vi "Refresh Channel Pairing.vi"(8 "error in (no error)":errorcluster, 10 "engine configuration in":refnum<class "engine configuration.lvclass">, 11 "E2E editor node in":refnum<class "E2E Tag Exchange editor node.lvclass">) -> (0 "error out":errorcluster, 2 "engine configuration out":refnum<class "engine configuration.lvclass">, 3 "E2E editor node out":refnum<class "E2E Tag Exchange editor node.lvclass">)   [LabVIEW 2015, in "E2E Tag Exchange editor node.lvclass"]
uses:
  E2E Tag Exchange editor node.lvclass
  <vilib>/NI/Module Execution Interface/Engine Configuration/engine configuration.lvclass
  E2E Tag Exchange editor node.lvclass/E2E Tag Exchange editor node.ctl
  module/configuration/E2E Tag Exchange configuration.lvclass/E2E Tag Exchange configuration.ctl
  <vilib>/NI/Configuration Framework/serializable configuration/NISE_CEF_serializable configuration.lvclass/NISE_CEF_serializable configuration.ctl
  module/configuration/Write Paired Module UID.vi
  module/configuration/Read Paired Module UID.vi
  <vilib>/Utility/LVClass/Get LV Class Name.vi
  <vilib>/NI/Configuration Framework/error generator/NISE_error generator.vi
  <vilib>/NI/DCAF/Tag Editor Core/Configuration Editor/Classes/Module editor node/module editor node.lvclass
  module/configuration/E2E Tag Exchange configuration.lvclass
  <vilib>/NI/Configuration Framework/serializable configuration/NISE_CEF_serializable configuration.lvclass
  <vilib>/NI/DCAF/Tag Editor Core/Configuration Editor/Classes/Engine Parent/Engine Parent Editor Node.lvclass
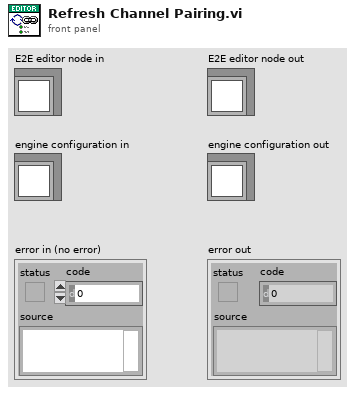
[diagram p1: front panel]
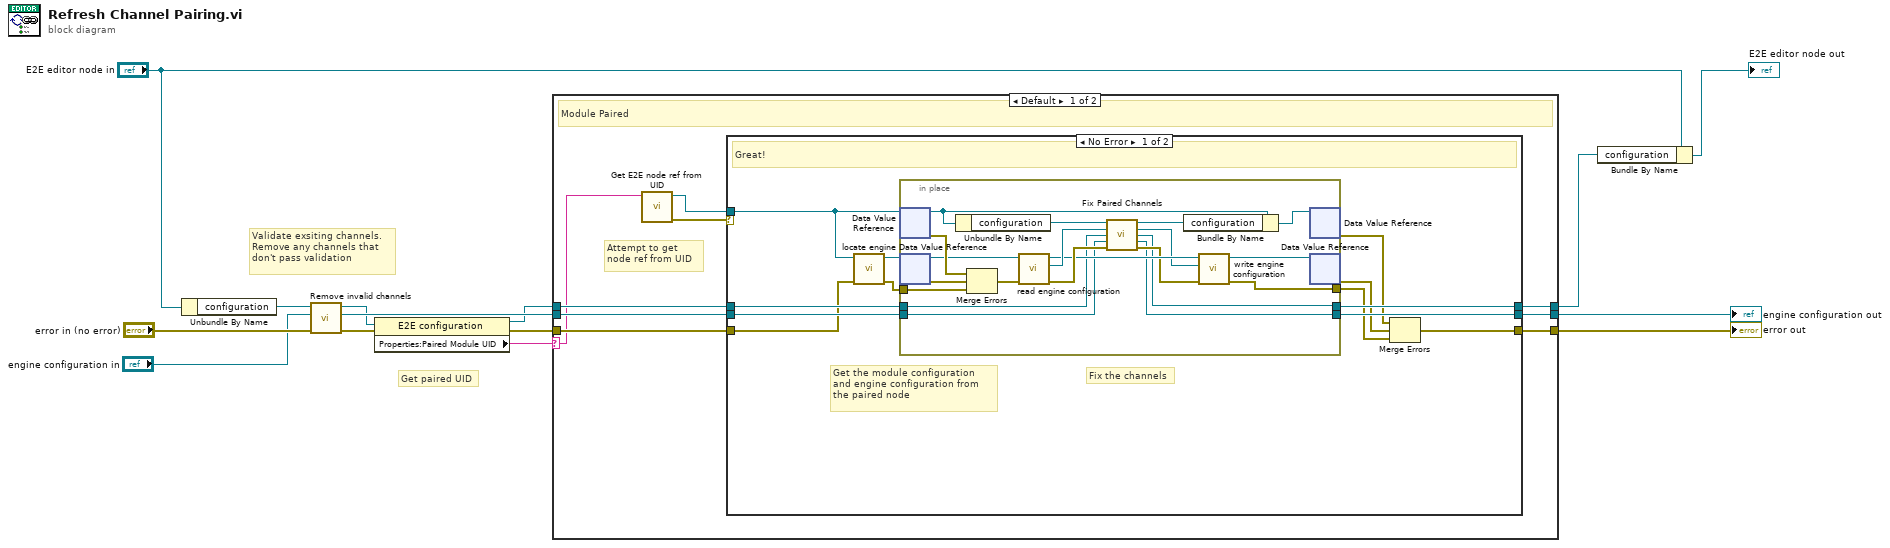
[diagram p0: block diagram]
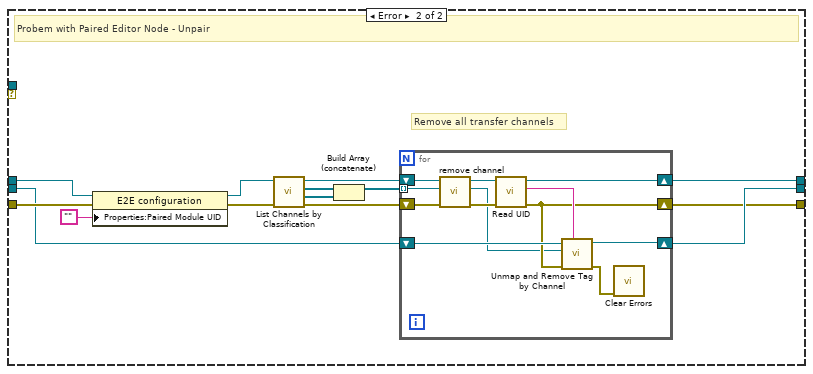
[diagram p2: hidden frame]
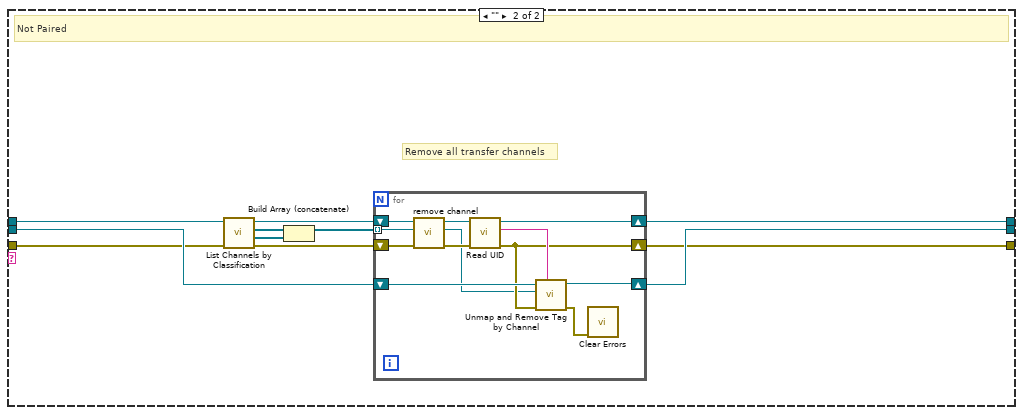
[diagram p3: hidden frame]
diagram:
  # "Get paired UID"
  # "Validate exsiting channels.\nRemove any channels that \ndon't pass validation"
  n1 = Unbundle By Name("E2E editor node in") -> ("configuration"=w14:refnum<class "E2E Tag Exchange configuration.lvclass">)
  n2 = call "Remove invalid channels.vi"("error in (no error)"="error in (no error)", "engine configuration in"="engine configuration in", "E2E configuration in"=w14) -> ("error out"=w11:errorcluster, "engine configuration out"=w8:refnum<class "engine configuration.lvclass">, "E2E configuration out"=w7:refnum<class "E2E Tag Exchange configuration.lvclass">)  [unwired: 6 in]
  n3 = property class="E2E configuration"(reference=w7, error in=w11) -> (reference out=w6:refnum<class "E2E Tag Exchange configuration.lvclass">, error out=w9:errorcluster, "Properties:Paired Module UID"=w10:string)
  n4 = case shown="Default" w10 {
    selector: w10 -> [w18 _]
    tunnel: w9 -> [w22 w81]
    tunnel: w8 -> [w20 w89]
    tunnel: w6 -> [w19 w85]
    tunnel: [w17 w87] -> w5
    tunnel: [w16 w88] -> w1
    tunnel: [w15 w86] -> w2
    frame Default {
      # "Attempt to get\nnode ref from UID"
      # "Module Paired"
      n5 = call "Get E2E node ref from UID.vi"("UID"=w18) -> ("error out"=w23:errorcluster, "E2E editor node ref"=w21:refnum<data-value>)  [unwired: 9 in]
      n6 = case shown="No Error" w23 {
        tunnel: w22 -> [w31 w68]
        tunnel: w21 -> [w33 _]
        tunnel: w20 -> [w35 w58]
        tunnel: w19 -> [w34 w67]
        tunnel: [w28 w56] -> w15
        tunnel: [w30 w60] -> w17
        tunnel: [w29 w57] -> w16
        frame No Error {
          # "Fix the channels"
          # "Get the module configuration\nand engine configuration from\nthe paired node"
          # "Great!"
          n7 = call <vilib>:"locate engine.vi"("error in"=w31, "component"=w33) -> ("error out"=w24:errorcluster, "engine"=w32:refnum<data-value>)  [unwired: 8 in]
          n8 = in-place {
            in-place-border: w35 -> [w41]
            in-place-border: w34 -> [w42]
            in-place-border: [w36] -> w27
            in-place-border: [w39] -> w30
            in-place-border: [w40] -> w29
            in-place-border: w24 -> [w55]
            n9 = in-place-dvr #1(w33) -> (w45:refnum<class "E2E Tag Exchange editor node.lvclass">, w53:errorcluster)
            n10 = in-place-dvr #2(w32) -> (w52:refnum<class "Engine Parent Editor Node.lvclass">, w54:errorcluster)
            n11 = Unbundle By Name(w45) -> ("configuration"=w49:refnum<class "E2E Tag Exchange configuration.lvclass">)
            n12 = Merge Errors(w53, w54, w55) -> (w51:errorcluster)
            n13 = call <vilib>:"read engine configuration.vi"("error in"=w51, "Engine Parent Editor Node in"=w52) -> ("error out"=w50:errorcluster, "engine configuration"=w48:refnum<class "engine configuration.lvclass">, "Engine Parent Editor Node out"=w47:refnum<class "Engine Parent Editor Node.lvclass">)  [unwired: 7 in]
            n14 = call "Fix Paired Channels.vi"("Paired E2E configuration in"=w49, "Paired engine configuration in"=w48, "E2E configuration in"=w42, "engine configuration in"=w41, "error in (no error)"=w50) -> ("Paired E2E configuration out"=w44:refnum<class "E2E Tag Exchange configuration.lvclass">, "Paired engine configuration out"=w46:refnum<class "engine configuration.lvclass">, "E2E configuration out"=w39:refnum<class "E2E Tag Exchange configuration.lvclass">, "engine configuration out"=w40:refnum<class "engine configuration.lvclass">, "error out"=w43:errorcluster)  [unwired: 6 in]
            n15 = Bundle By Name(cluster=w45, "configuration"=w44) -> (w38:refnum<class "E2E Tag Exchange editor node.lvclass">)
            n16 = call <vilib>:"write engine configuration.vi"("error in"=w43, "engine configuration"=w46, "Engine Parent Editor Node in"=w47) -> ("error out"=w36:errorcluster, "Engine Parent Editor Node out"=w37:refnum<class "Engine Parent Editor Node.lvclass">)  [unwired: 7 in]
            n17 = in-place-dvr #1(w38) -> (w25:errorcluster)  [unwired: 1 out]
            n18 = in-place-dvr #2(w37) -> (w26:errorcluster)  [unwired: 1 out]
          }
          n19 = Merge Errors(w25, w26, w27) -> (w28:errorcluster)
        }
        frame Error {
          # "Remove all transfer channels"
          # "Probem with Paired Editor Node - Unpair"
          n20 = property class="E2E configuration"(reference=w67, error in=w68, "Properties:Paired Module UID"="") -> (reference out=w61:refnum<class "E2E Tag Exchange configuration.lvclass">, error out=w59:errorcluster)
          n21 = call "List Channels by Classification.vi"("E2E configuration in"=w61) -> ("Output Channels"=w63:refnum<class "TBM channel.lvclass">[], "Input Channels"=w64:refnum<class "TBM channel.lvclass">[], "E2E configuration out"=w65:refnum<class "E2E Tag Exchange configuration.lvclass">)  [unwired: 8 in]
          n22 = Build Array (concatenate)(w64, w63) -> (w62:refnum<class "TBM channel.lvclass">[])
          n23 = for {
            tunnel: w62 -> [w74] mode=indexing
            shift-right: [w75] -> w60
            shift-left: w65 -> [w80]
            shift-right: [w76] -> w57
            shift-left: w58 -> [w77]
            shift-right: [w71] -> w56
            shift-left: w59 -> [w73]
            n24 = call "remove channel.vi"("error in (no error)"=w73, "channel"=w74, "E2E configuration in"=w80) -> ("error out"=w72:errorcluster, "removed channel"=w70:refnum<class "TBM channel.lvclass">, "E2E configuration out"=w79:refnum<class "E2E Tag Exchange configuration.lvclass">)  [unwired: 6 in]
            n25 = call <vilib>:"Read UID.vi"("error in"=w72, "configuration in"=w79) -> ("error out"=w71:errorcluster, "instance id"=w78:string, "configuration out"=w75:refnum<class "E2E Tag Exchange configuration.lvclass">)  [unwired: 7 in]
            n26 = call "Unmap and Remove Tag by Channel.vi"("owner ID"=w78, "error in"=w71, "channel"=w70, "engine configuration in"=w77) -> ("error out"=w69:errorcluster, "engine configuration out"=w76:refnum<class "engine configuration.lvclass">)  [unwired: 6 in]
            n27 = call <vilib>:"Clear Errors.vi"("error in (no error)"=w69) -> ()  [unwired: 5 in, 2 out]
          }
        }
      }
    }
    frame "" {
      # "Remove all transfer channels"
      # "Not Paired"
      n28 = call "List Channels by Classification.vi"("E2E configuration in"=w85) -> ("Output Channels"=w83:refnum<class "TBM channel.lvclass">[], "Input Channels"=w84:refnum<class "TBM channel.lvclass">[], "E2E configuration out"=w90:refnum<class "E2E Tag Exchange configuration.lvclass">)  [unwired: 8 in]
      n29 = Build Array (concatenate)(w84, w83) -> (w82:refnum<class "TBM channel.lvclass">[])
      n30 = for {
        tunnel: w82 -> [w96] mode=indexing
        shift-right: [w97] -> w87
        shift-left: w90 -> [w102]
        shift-right: [w98] -> w88
        shift-left: w89 -> [w99]
        shift-right: [w93] -> w86
        shift-left: w81 -> [w95]
        n31 = call "remove channel.vi"("error in (no error)"=w95, "channel"=w96, "E2E configuration in"=w102) -> ("error out"=w94:errorcluster, "removed channel"=w92:refnum<class "TBM channel.lvclass">, "E2E configuration out"=w101:refnum<class "E2E Tag Exchange configuration.lvclass">)  [unwired: 6 in]
        n32 = call <vilib>:"Read UID.vi"("error in"=w94, "configuration in"=w101) -> ("error out"=w93:errorcluster, "instance id"=w100:string, "configuration out"=w97:refnum<class "E2E Tag Exchange configuration.lvclass">)  [unwired: 7 in]
        n33 = call "Unmap and Remove Tag by Channel.vi"("owner ID"=w100, "error in"=w93, "channel"=w92, "engine configuration in"=w99) -> ("error out"=w91:errorcluster, "engine configuration out"=w98:refnum<class "engine configuration.lvclass">)  [unwired: 6 in]
        n34 = call <vilib>:"Clear Errors.vi"("error in (no error)"=w91) -> ()  [unwired: 5 in, 2 out]
      }
    }
  }
  "error out" <- w2
  "engine configuration out" <- w1
  n35 = Bundle By Name(cluster="E2E editor node in", "configuration"=w5) -> (→"E2E editor node out":refnum<class "E2E Tag Exchange editor node.lvclass">)
